vi "MainGui.vi"() -> ()   [LabVIEW 2016]
uses:
  MainGui.TestOptionsGui.ctl
  MainGui.TopBar.ctl
  tools/TouchPanel/TouchPanel.Keyboard.ctl
  tools/EventLog/EventLog.Gui.Sets.ctl
  tools/EventLog/EventLog.EventLevelOperatorGui.ctl
  MainGui.Action.ctl
  Sequence/Sequence.MainMode.ctl
  Station/Station.SwButtons.Fglb.Action.ctl
  Sequence/Sequence.UserAction.ctl
  MainGui.UserMsg.ctl
  tools/Translator/Translator.Message.ctl
  <vilib>/Utility/miscctls.llb/LVRowAndColumnTypeDef.ctl
  <vilib>/Utility/miscctls.llb/LVRowAndColumnUnsignedTypeDef.ctl
  tools/User/User.Level.ctl
  tools/CitTemplate/citTemplate.errData.ctl
  tools/EventLog/EventLog.EventSource.ctl
  Drivers/FestoCPX/FestoCPX.State.ctl
  Drivers/V7310/V7310.Data.Status.State.ctl
  Drivers/Keyence/Keyence.Data.Status.State.ctl
  tools/Translator/Translator.FormatMessage.vi
  tools/Config/Config.Global.vi
  Global/ApplicationGlobal.vi
  Station/Station.Global.vi
  tools/Translator/Translator.Global.vi
  Drivers/Keyence/LowLevel/Keyence.Global.vi
  Drivers/FestoCPX/FestoCPX.Global.vi
  Drivers/V7310/LowLevel/V7310.Global.vi
  <vilib>/Utility/inputDevices.llb/closeMouse.vi
  tools/User/User.Global.vi
  Database/Database.Global.vi
  MainGui.ButtonType.ctl
  <vilib>/Utility/miscctls.llb/LVRectTypeDef.ctl
panel:
  in  "Btn_ScannerGui":bool
  in  "Btn_Stats":bool
  in  "Btn_SelectPlate":bool
  in  "Btn_Scan":bool
  in  "Btn_DoorLock":bool
  in  "Btn_Reject":bool
  in  "Btn_Start":bool
  in  "Btn_ManualView":bool
  in  "Btn_Lock":bool
  in  "Btn_Pause":bool
  in  "Btn_Results":bool
  in  "Btn_Accept":bool
  in  "Btn_Next":bool
  in  "Btn_Exit":bool
  in  "Btn_Order":bool
  in  "Btn_Logs":bool
  in  "Btn_Base":bool
  in  "Btn_Manual":bool
  in  "Btn_Process":bool
  in  "Btn_Stop":bool
  in  "Btn_Mode":bool
  out "~ModeInUse":bool
  in  "EmptyButtons":bool[](array[boolean])
  out "Panel":refnum<vi>
  out "SelectModeTS":timestamp
  out "BlinkIndicator":bool
  out "RefNoTimer":timestamp
  out "Btns":refnum<vi>[](array[refnum])
  in  "TopBarTab":enum32{"Status", "Manual", "Logs", "Error"}(tab)=enum."Logs"
  out "StatusMsg":string
  in  "TestOptions":T1
  in  "EventModeOptions":T2={"IncludeBegin"=FALSE, "dtm_Begin"=timestamp(0 s since 1904-01-01), "IncludeEnd"=FALSE, "dtm_End"=timestamp(0 s since 1904-01-01), "Events Level Operator"=enum.">=", "Level"=1, "Source"=1, "SearchText"="", "Freeze"=FALSE} caption="Event.Sets" {"Source" items=["All", "Gui", "Ref", "File", "Arch", "Seq", "CPX", "DB", "Laser", "Scan.P", "Scan.O"]; "Level" items=["ALL", "Debug", "Info", "Warning", "Błąd"]; "dtm_End" format="%<%.1X\n%x>T"; "dtm_Begin" format="%<%.1X\n%x>T"}
  out "ErrMsg":i32(listbox)
  in  "Btn_ErrConfirm":bool
  in  "TopBar":T4={"~touchpanel"=FALSE, "_loop"=4, "_ver"="", "_flag"=bytes[0], "time"="", "Btn_ShowErr"=FALSE, "DB"=FALSE, "CPX"=FALSE, "LSR"=FALSE, "SCAN"=FALSE, "SCAN 2"=FALSE}
  in  "start here":bool
  out "MainPanelViRef":refnum<vi>
  out "DeviceID":refnum<k1> caption="device ID"
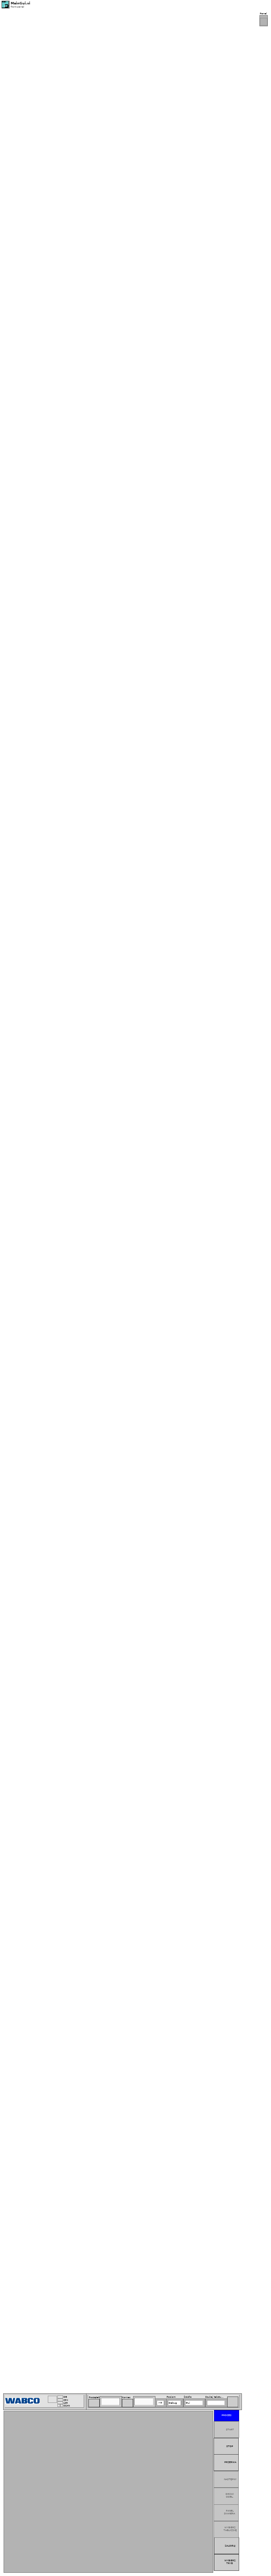
[diagram p1: front panel]
types:
  T1 = typedef "MainGui.TestOptionsGui.ctl" = cluster{"IgnoreResults":bool, "IgnoreImages":bool, "Service":bool}
  T2 = typedef "EventLog.Gui.Sets.ctl" = cluster{"IncludeBegin":bool, "dtm_Begin":timestamp, "IncludeEnd":bool, "dtm_End":timestamp, "Events Level Operator":T3, "Level":u16, "Source":u16, "SearchText":string, "Freeze":bool}
  T3 = typedef "EventLog.EventLevelOperatorGui.ctl" = enum16{">=", "=", "<="}
  T4 = typedef "MainGui.TopBar.ctl" = cluster{"~touchpanel":T5, "_loop":i32, "_ver":string, "_flag":picture, "time":string, "Btn_ShowErr":bool, "DB":bool, "CPX":bool, "LSR":bool, "SCAN":bool, "SCAN 2":bool}
  T5 = typedef "TouchPanel.Keyboard.ctl" = bool
  T6 = enum8{"Enabled", "Disabled", "Disabled and Grayed Out"}
  T7 = typedef "Translator.Message.ctl" = enum16{"-", "Event confirmed", "Log out", "Log in", "Shutdown", "Cancel", "Start", "Begin time", "End time", "Duration", "Service Mode", "Ignore Results", "Serial Format", "On", "Off", "OK", "NOK", "NOK %s", "Home", "Work", "Close", "Open", "In progress...", "Missing", "Empty", "Hardware failure", "Initial", "Default", "Total", "Out of range", "Free disk space is below 1GB - contact technician", "Error %d >> %s", "Error %d >> %s >> %s", "Msg %d >> %s", "Laser msg %d %s", "Laser cmd error %s %d", "Laser cmd failed %s", "Laser cmd warning %s", "Laser disconnected", "Laser status %s", "Laser already started", "Laser job unkonwn %s", "Laser job missing %s", "Laser job select failure %s", "Unable to start laser printing (%s)", "Unable to stop laser printing (%s)", "Laser marking aborted", "Laser marking timeout", "Unable to reset Laser Interlock (%s)", "Unable to trigger Laser. Laser not ready (%s)", "Laser job '%s' coordinates not configured", "Starting %s", "Quitting %s", "Configured", "Initializing", "Quitting", "Loading", "Loaded %d results", "Loaded %d events", "Running", "Stopped", "Summary", "Laser", "Do you want to continue?", "Do you want to delete the configuration?", "The configuration is being used by an order. Unable to delete!", "Press confirm button", "Station is not based. Do you want to exit?", "Station requires changeover. Do you want to run the test?", "Test options are not set as default. Do you want to continue?", "Formatting of WabcoNo is disabled. Do you want to continue?", "Product not detected. Do you want to continue?", "Product scan failed. Do you want to continue?", "Calibration", "Log out?", "System", "All", "IDLE", "Translating...%s", "Not found", "Alarm %s", "Run", "Skip", "Abort", "Repeat", "Please wait...", "Database disconnected", "Database disconnected - changeover disabled!", "Login to database successful", "Login to database failed: %d; %s", "Unable to check the product status of reference %d - database disconnected", "Unable to set the product status of reference %d - database disconnected", "Variant file backup %s", "Read variant (%s)", "Result", "Station armed!", "Station requires changeover!", "Select reference number...", "EMERGENCY BUTTON - press Control button", "EMERGENCY DOOR - press Control button", "Resetting Emergency...", "Unable to reset safety circuit - Emergency Button pressed", "Unable to reset safety circuit - Emergency Side Door open", "Station not based", "Station based", "Station not empty", "Station basing...", "No order", "Press Start to begin new order", "Scanning new order", "Order NOK. Correct or scan again", "Order OK. Press Accept", "Order ready", "Revolver incorrect", "Fork incorrect", "Revolver missing", "Revolver empty", "Container missing", "Offline results", "Offline statistics", "Updating statistics %.1f %%", "DMC Configurator", "Door open", "Close the front door", "Press start button", "Done. Open the front door", "Running...", "Running...%.1f %%", "Pause %s", "Pause %s. NOK container missing", "Pause %s. OK container missing", "Pause %s. Revolver empty", "Pause %s. Revolver missing", "Pause %s. Revolver incorrect", "Pause %s. Fork missing", "Pause %s. Fork incorrect", "Pause %s. Too many failures", "Pause %s. Unloading failure", "Pause %s. One slot is not working", "Pause %s. Part order is done. Empty OK container", "Pause %s. Unable to move product to slot", "Pause %s. Unable to move back product pusher", "Pause %s. Unable to lift product", "Pause %s. Unable to move back product lifter", "Pause %s. Unable to move product arm to Work", "Pause %s. Unable to move product arm to NOK", "Pause %s. Unable to move product arm to OK", "Pause %s. Unable to unsuck the NOK product", "Pause %s. Unable to drop the NOK product", "Pause %s. Product OK missing", "Pause %s. Unable to unsuck the OK product", "Pause %s. Unable to drop the OK product", "Stopping...", "File '%s' is missing", "File '%s' is broken", "File '%s' is running", "Log file started (%s)", "Log file ended (%s)", "Log file stopped (%s)", "Log file ignored (%s)", "Log file exported (%s)", "Log file export failed (%s)", "Wrong serial number in log file", "Wrong reference number in log file", "Test steps are missing", "%s = %.3f", "Process param '%s' not found in DB", "Process param '%s' wrong order", "Process param '%s' value %.3f out of limits (%.3f; %.3f)", "Step%d param '%s' not found in DB", "Step%d param '%s' wrong order", "Step%d param '%s' value %.3f out of limits (%.3f; %.3f)", "Step%d EV '%s' not found in DB", "Step%d EV '%s' wrong order", "\"%s\" not found in DB", "\"%s\" wrong order", "\"%s\" value %.3f out of limits (%.3f; %.3f)", "\"%s\" not found in software", "Process init (%s)", "Process started", "Process restarted", "Process run", "Process done", "Process done - remove OK container", "Process aborted", "Process aborted at work", "Process aborted at home", "Process error", "Process error at home", "Process error at work", "Process close", "Process pause", "Process continue", "Process door open", "Process door close", "Process pause at slot %s due to %s", "Select plate from the order to process", "Do you want to start the process?", "Do you want to continue the process?", "There is unfinished order. Do you want to put the new order?", "Product %s %d OK", "Product %s %d NOK", "Unable to unload the slot %s. Product missing in the slot", "Unable to unload the slot %s. Product already in the arm", "Unable to accept the product as OK. Product missing in slot %s", "Unable to accept the product as OK. Product could not drop into the container at slot %s", "Unable to accept the product as NOK. Product could not drop into the container at slot %s", "Scan failed. Error %s", "Scan failed. Scanner disconnected", "Scan failed. Wrong Wabco number %d, limit (%d,%d)", "Scan failed. Wrong serial number %d, limit (%d,%d)", "Scan failed. Wrong date %d, limit (%d,%d)", "Scan failed. Wrong product wabco number %d (expected %d)", "Scan failed. Wrong product serial number %d (expected > 0)", "Scan OK %s", "Scan failed. Unable to determine table position (%s)", "Scan failed. Timeout", "Tune failed. Scanner disconnected", "Tune failed. Timeout", "%s = %d", "%s = %d->%d", "Unable to set %s = %.2f - Air Pressure Inside off", "Unable to set digital output '%s' = %d", "Unable to activate air pressure inside - timeout", "Unable to activate air pressure inside - aborted", "Unable to switch on Air Main Valve - Air Pressure Inlet off", "Unable to switch on Air Main Valve - Door open", "Unable to switch off Air Main Valve - timeout", "Unable to switch off Air Main Valve - aborted", "Unable to rotate Table - timeout", "Unable to rotate Table - aborted", "Unable to rotate Table - Product Move not in Home position", "Unable to rotate Table - Air Pressure Inside off", "Unable to rotate Table - Product Lift A not in Home position", "Unable to rotate Table - Product Lift B not in Home position", "Unable to rotate Table - unlock before movement timeout", "Unable to rotate Table - lock after movement timeout", "Unable to move Table Lock to %s position - timeout", "Unable to move Table Lock to %s position - aborted", "Unable to move Table Lock to %s position - Air Pressure Inside off", "Unable to move Table Lock to %s position - Table not in position", "Unable to move Product Lift A to %s position - timeout", "Unable to move Product Lift B to %s position - timeout", "Unable to move Product Lift A to %s position - aborted", "Unable to move Product Lift B to %s position - aborted", "Unable to move Product Lift A to %s position - Air Pressure Inside off", "Unable to move Product Lift B to %s position - Air Pressure Inside off", "Unable to move Product Lift A to %s position - Table not locked", "Unable to move Product Lift B to %s position - Table not locked", "Unable to move Product Lift A to %s position - Product Arm not in Work position", "Unable to move Product Lift B to %s position - Product Arm not in Work position", "Unable to set Product Suction Gripper %s to %s - timeout", "Unable to set Product Suction Gripper %s to %s - aborted", "Unable to set Product Suction Gripper %s to %s - Air Pressure Inside off", "Unable to set Product Suction Gripper %s to %s - Table slot unkown", "Unable to move Product Arm to %s position - timeout", "Unable to move Product Arm to %s position - aborted", "Unable to move Product Arm to %s position - Air Pressure Inside off", "Unable to move Product Arm to %s position - Product Lift A not in Home position", "Unable to move Product Arm to %s position - Product Lift B not in Home position", "Unable to move Product to %s position - timeout", "Unable to move Product to %s position - aborted", "Unable to move Product to %s position - Air Pressure Inside off", "Unable to move Product to %s position - Table not in position"}
  T8 = typedef "Sequence.MainMode.ctl" = enum16{"Process", "Base", "Order", "Manual", "Logs", "Results", "Stats", "DMC Config"}
  T9 = typedef "Station.SwButtons.Fglb.Action.ctl" = enum16{"get", "start", "stop", "control"}
  T10 = typedef "Sequence.UserAction.ctl" = enum16{"-", "Stop", "Pause", "Continue", "Next"}
  T11 = typedef "LVRectTypeDef.ctl" = cluster{"Left":i16, "Top":i16, "Right":i16, "Bottom":i16}
  T12 = enum32{"Invalid", "Standard", "Closed", "Hidden", "Minimized", "Maximized"}
  T13 = typedef "MainGui.UserMsg.ctl" = cluster{"Msg":T7, "Arguments":variant[], "BgColor":u32, "TxtColor":u32, "Blink":bool}
  T14 = enum32{"invalid app kind", "Development System", "Run Time System", "Student Edition", "Embedded LabVIEW", "Evaluation", "Custom"}
  T15 = typedef "LVRowAndColumnUnsignedTypeDef.ctl" = cluster{"Row":u32, "Column":u32}
  T16 = typedef "LVRowAndColumnTypeDef.ctl" = cluster{"Row":i32, "Column":i32}
  T17 = typedef "User.Level.ctl" = enum16{"-", "Operator", "Technician", "Administrator"}
  T18 = typedef "citTemplate.errData.ctl" = cluster{"ts":timestamp, "src":T19, "instance":i32, "action":string, "error":errorcluster, "unconfirmed":bool}
  T19 = typedef "EventLog.EventSource.ctl" = enum16{"All", "Gui", "Ref", "File", "Arch", "Seq", "CPX", "DB", "Laser", "Scan.P", "Scan.O"}
  T20 = typedef "Keyence.Data.Status.State.ctl" = enum16{"First", "Init", "Reset", "Idle", "Scan", "Tune"}
  T21 = typedef "V7310.Data.Status.State.ctl" = enum16{"First", "Init", "Msg", "Error", "Abort", "Idle", "Run"}
  T22 = typedef "FestoCPX.State.ctl" = enum16{"First", "Error", "Init", "Run"}
  T23 = typedef "MainGui.Action.ctl" = enum32{"idle", "constructor", "destructor", "--- MainGui ---", "Error.Update", "Error.Confirm", "Buttons.Update", "Mode.Select", "Mode.Select.Seq", "Status.Update", "TopBar.Update"}
  T24 = typedef "Station.Data.ctl" = cluster{"State":T25, "Seq.State":T26, "Seq.BreakReason":T27, "Seq.BreakSource":T28, "Hw failure":bool, "Unconfirmed":bool, "Station empty":bool, "Home err":bool, "Order done":bool, "DUT present":T29, "EmgState":T30, "Sets":T31, "StatusBits":T33}
  T25 = typedef "Station.State.ctl" = enum16{"Idle", "Ready", "Run", "Stop", "Error", "Home", "Done", "Emg"}
  T26 = typedef "Sequence.State.ctl" = enum16{"Init", "Idle", "Home", "Work", "Run", "Pause"}
  T27 = typedef "Sequence.Test.BreakReason.ctl" = enum16{"-", "NOK container", "OK container", "Rev empty", "Rev missing", "Rev wrong", "Fork missing", "Fork wrong", "NOK limit", "Unload failure", "Single slot", "Part done", "Err: Prod move work", "Err: Prod move home", "Err: Prod lift work", "Err: Prod lift home", "Err: Prod Arm Work", "Err: Prod Arm NOK", "Err: Prod Arm OK", "Err: Prod NOK suck", "Err: Prod NOK drop", "Err: Prod OK missing", "Err: Prod OK suck", "Err: Prod OK drop"}
  T28 = typedef "Sequence.Test.BreakSource.ctl" = enum16{"-", "A", "B", "A/B"}
  T29 = typedef "FestoCPX.Station.ProdPresent.ctl" = cluster{"Slot1":cluster{"A":bool, "B":bool}, "Slot2":cluster{"A":bool, "B":bool}, "Slot3":cluster{"A":bool, "B":bool}, "Slot4":cluster{"A":bool, "B":bool}, "Final":cluster{"A":bool, "B":bool}, "OK":cluster{"A":bool, "B":bool}, "Container":cluster{"OK":bool, "NOK":bool}}
  T30 = typedef "FestoCPX.Station.EmgState.ctl" = cluster{"Button":bool, "SideDoor":bool, "FrontDoor":bool, "DoorSecured":bool}
  T31 = typedef "Sequence.UserData.ctl" = cluster{"GuiMode":T8, "Test":T32, "ContinueOrder":bool}
  T32 = typedef "MainGui.TestOptions.ctl" = cluster{"IgnoreResults":bool, "IgnoreImages":bool, "ServiceMode":bool}
  T33 = typedef "Station.Home.Status.Bits.ctl" = cluster{"Door Close":bool, "Rev OK":bool, "Fork OK":bool, "Container OK":bool, "Station empty":bool}
  T34 = typedef "Sequence.PlateType.ctl" = enum16{"Wabco", "Client"}
  T35 = typedef "LVPositionTypeDef.ctl" = cluster{"Left":i32, "Top":i32}
  T36 = typedef "Keyence.Data.Status.ctl" = cluster{"State":T20, "Ref":refnum<k5>, "Bank":u8, "Version":string, "Model":string, "EndTS":timestamp, "ImgPath":path, "Tuned":bool}
  T37 = typedef "FestoCPX.Data.Status.ctl" = cluster{"State":T22, "Conn":refnum<k5>, "TS":timestamp}
  T38 = typedef "V7310.Data.Status.ctl" = cluster{"State":T21, "LaserStatus":T39, "LaserStatusRaw":string, "Ref":refnum<k5>, "RTC TS":timestamp, "Conn TS":timestamp, "Msg":T40[], "JobInUse":string, "Jobs":string[], "Vars":T41[]}
  T39 = typedef "V7310.LaserStatus.ctl" = enum16{"-", "FatalError", "Initialize", "KeySwitchOpen", "TimeoutInterlock", "InterlockOpen", "StartUp", "ShutterlockOpen", "Standby", "Ready", "PrepareForMarking", "WaitForTrigger", "Marking"}
  T40 = typedef "V7310.Message.Data.ctl" = cluster{"ID":i32, "Msg":string}
  T41 = typedef "V7310.Job.Variable.ctl" = cluster{"Name":string, "Value":string}
  T42 = typedef "Database.Main.Data.Status.ctl" = cluster{"Run":bool, "Handle":i32, "ConnTS":timestamp, "DbTime":timestamp, "DbTimeCode":dbl, "DbTimeOffset":dbl}
  T43 = typedef "MainGui.ButtonType.ctl" = enum32{"Exit", "Mode", "Process", "Base", "Order", "Manual", "Logs", "Results", "Accept", "Reject", "Start", "Stop", "Next", "Pause", "Lock", "ManualView", "DoorLock", "Scan", "Select", "ScannerGui", "Stats"}
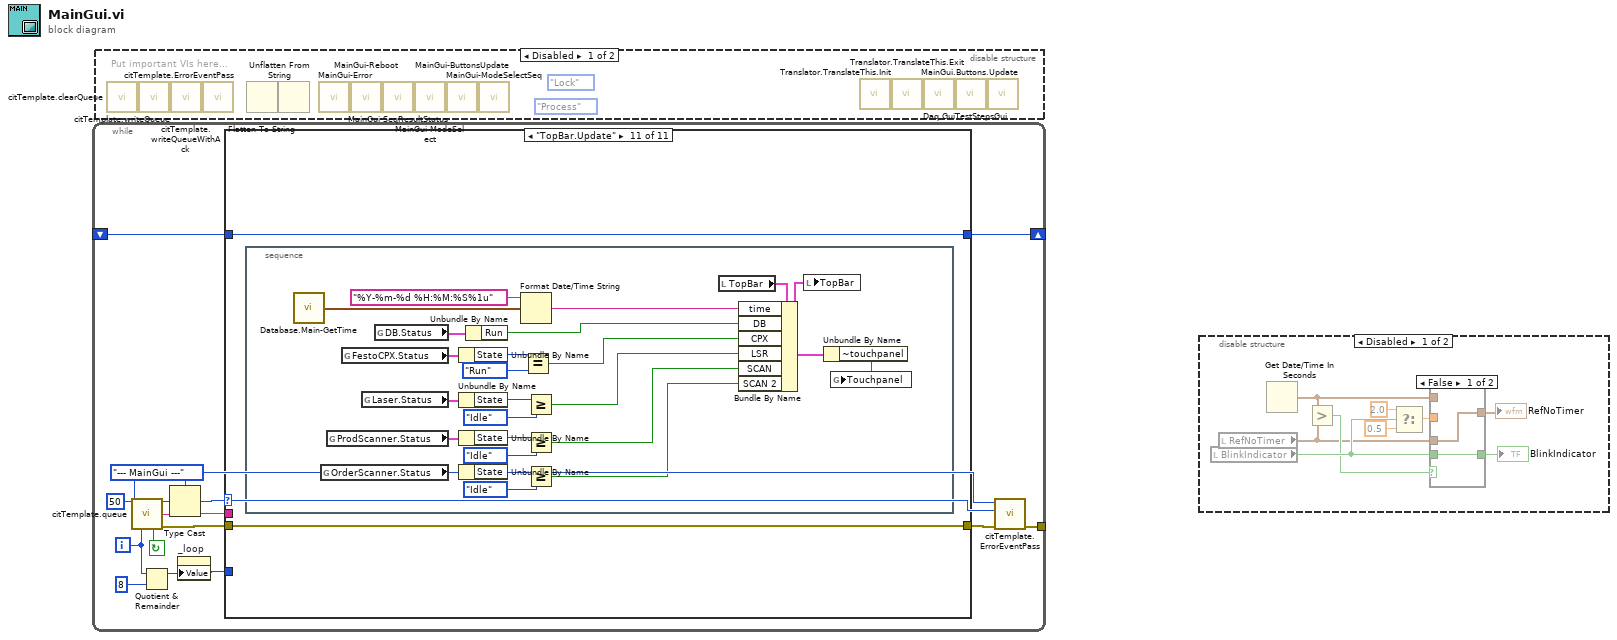
[diagram p0: block diagram]
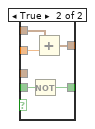
[diagram p2: hidden frame]
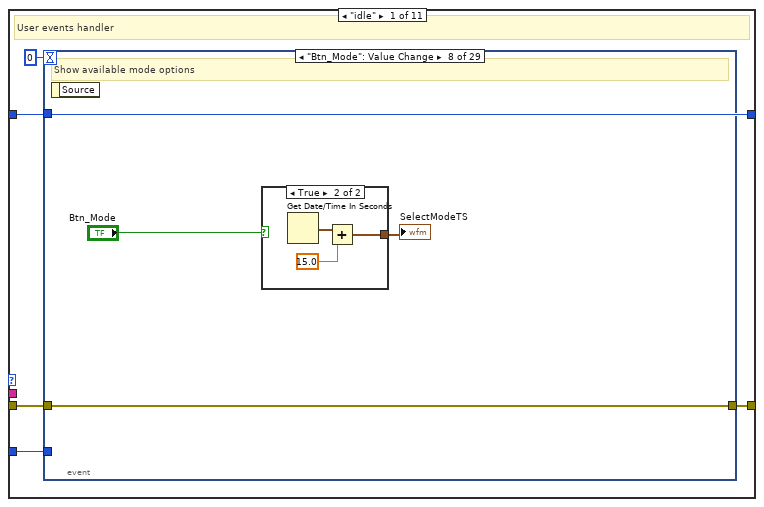
[diagram p5: hidden frame]
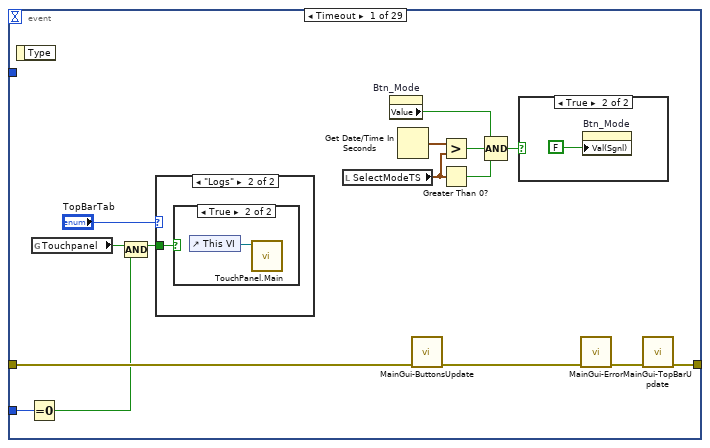
[diagram p6: hidden frame]
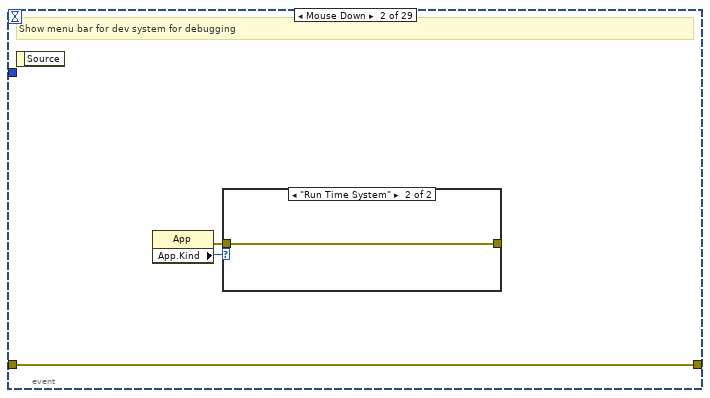
[diagram p10: hidden frame]
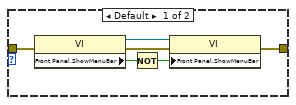
[diagram p11: hidden frame]
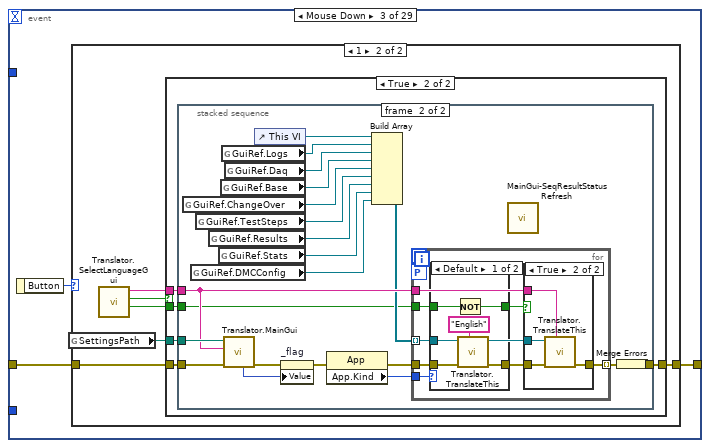
[diagram p12: hidden frame]
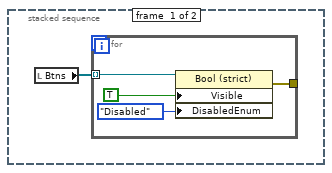
[diagram p15: hidden frame]
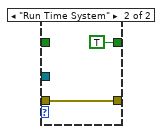
[diagram p17: hidden frame]
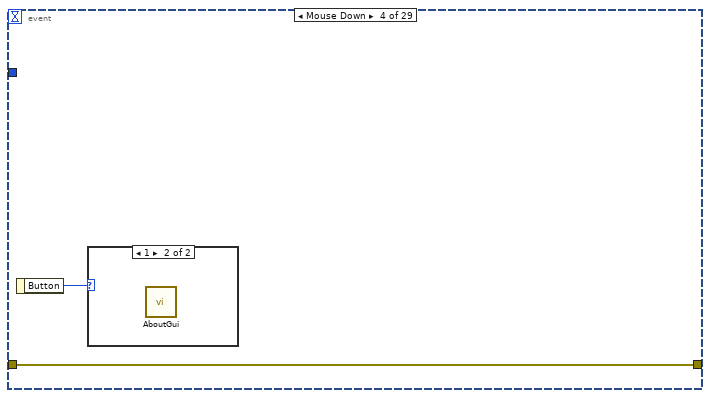
[diagram p18: hidden frame]
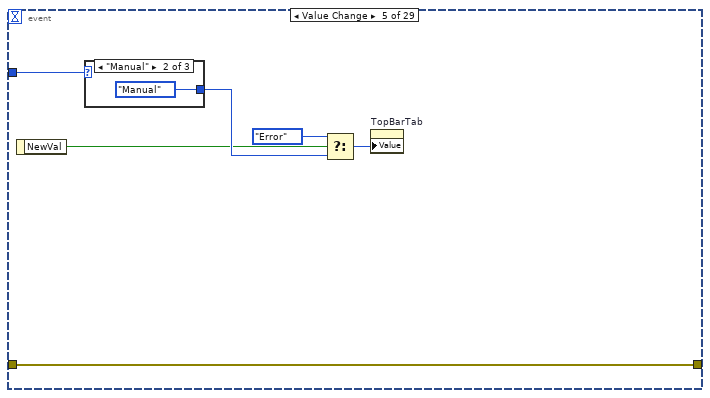
[diagram p20: hidden frame]
diagram:
  n1 = while {
    tunnel: [w7] -> _
    shift-right: [w2] -> _
    shift-left: _ -> [w4]
    i -> [w8]
    stop <- w11 continue-if-true
    w10 = MainGui.Action."--- MainGui ---" ("Action")
    n2 = call "citTemplate.queue.vi"("ms timeout (250 ms)"=50, "event enum"=w10, "iteration (-1)"=w8) -> ("event out"=w14:u32, "(flatten) data out"=w13:string, "continue"=w11:bool, "error out"=w12:errorcluster)  [unwired: 2 in, 7 out]
    n3 = Quotient & Remainder(x=w8, y=8) -> (x-y*floor(x/y)=w1:i32)  [unwired: 1 out]
    n4 = Type Cast(type=w10, x=w14) -> (*(type *) &x=w6:T23)
    n5 = property on="_loop" class="Ring (strict)"("Value"=w1) -> ()  [unwired: 2 in, 2 out]
    n6 = case shown="\"TopBar.Update\"" w6 {
      selector: w6 -> [_ _ _ w381 _ _ _ _ _ _ _]
      tunnel: w13 -> [_ _ _ w382 _ _ _ w444 _ w537 _]
      tunnel: w12 -> [w19 w247 w336 w384 w396 w426 w434 w445 w515 w538 w547]
      tunnel: w4 -> [w16 _ w334 w380 w393 w427 w437 w439 w516 w539 w548]
      tunnel: [w16 w246 w334 w380 w393 w427 w437 w440 w516 w539 w548] -> w2
      tunnel: [w18 w245 w335 w373 w397 w425 w432 w441 w510 w535 w547] -> w3
      tunnel: w1 -> [w15 _ _ _ _ _ _ _ _ _ _]
      frame "idle" {
        # "User events handler"
        n7 = event shown="[7] \"Btn_Mode\": Value Change" {
          selector: _ -> [_ _ _ _ _ _ _ _ _ _ _ _ _ _ _ _ _ _ _ _ _ _ _ _ _ _ _ _ _]
          dyn-events: _ -> [_ _ _ _ _ _ _ _ _ _ _ _ _ _ _ _ _ _ _ _ _ _ _ _ _ _ _ _ _]
          timeout: 0 -> [_ _ _ _ _ _ _ _ _ _ _ _ _ _ _ _ _ _ _ _ _ _ _ _ _ _ _ _ _]
          tunnel: w19 -> [w34 w40 w49 w112 w115 w124 w126 w146 w152 w155 w158 w161 w164 w167 w169 w173 w188 w196 w198 w201 w207 w209 w213 w214 w220 w237 w240 w242 w244]
          tunnel: [w33 w40 w48 w112 w115 w124 w125 w146 w151 w154 w156 w160 w163 w166 w168 w172 w186 w196 w197 w201 w206 w208 w212 w214 w220 w237 w239 w241 w244] -> w18
          tunnel: w16 -> [_ _ _ _ w118 _ _ _ _ _ _ _ _ _ _ w171 w187 _ _ _ _ _ _ _ w218 _ _ _ _]
          tunnel: w15 -> [w23 _ _ _ _ _ _ _ _ _ _ _ _ _ _ _ _ _ _ _ _ _ _ _ _ _ _ _ _]
          event Timeout {
            n8 = event-data() -> ()  [unwired: 1 in, 1 out]
            n9 = Equal To 0?(x=w23) -> (x = 0?=w21:bool)
            n10 = global read "Config.Global.vi" "Touchpanel"() -> (w32:bool)
            n11 = Compound Arithmetic op=AND(w32, w21) -> (w22:bool)
            n12 = case shown="\"Logs\"" "TopBarTab" {
              tunnel: w22 -> [_ w35]
              frame Default {
              }
              frame "Logs" {
                n13 = case shown="True" w35 {
                  frame False {
                  }
                  frame True {
                    n14 = control-ref of="This VI"() -> (w36:refnum<vi>)
                    n15 = call "TouchPanel.Main.vi"("VI ref"=w36) -> ()  [unwired: 8 in, 3 out]
                  }
                }
              }
            }
            n16 = local read "SelectModeTS"() -> (w25:timestamp)
            n17 = property on="Btn_Mode" class="Bool (strict)"() -> ("Value"=w28:bool)  [unwired: 2 in, 2 out]
            n18 = Get Date/Time In Seconds() -> (seconds since 1Jan1904=w24:timestamp)
            n19 = call "MainGui-ButtonsUpdate.vi"("error in (no error)"=w34) -> ("error out"=w30:errorcluster)  [unwired: 10 in]
            n20 = Greater?(x=w24, y=w25) -> (0:w26:bool)
            n21 = Greater Than 0?(x=w25) -> (x > 0?=w27:bool)
            n22 = Compound Arithmetic op=AND(w28, w26, w27) -> (w29:bool)
            n23 = case shown="True" w29 {
              frame False {
              }
              frame True {
                n24 = property on="Btn_Mode" class="Bool (strict)"("Val(Sgnl)"=FALSE ("Value (Signaling)")) -> ()  [unwired: 2 in, 2 out]
              }
            }
            n25 = call "MainGui-Error.vi"("error in (no error)"=w30) -> ("error out"=w31:errorcluster)  [unwired: 10 in]
            n26 = call "MainGui-TopBarUpdate.vi"("error in (no error)"=w31) -> ("error out"=w33:errorcluster)  [unwired: 10 in]
          }
          event Mouse Down {
            # "Show menu bar for dev system for debugging"
            n27 = event-data() -> ()  [unwired: 1 in, 1 out]
            n28 = property class="App"() -> (error out=w38:errorcluster, "App.Kind"=w39:T14)  [unwired: 2 in, 1 out]
            n29 = case shown="\"Run Time System\"" w39 {
              tunnel: w38 -> [w42 w47]
              tunnel: [w41 w47] -> _
              frame Default {
                n30 = property class="VI"(error in=w42) -> (reference out=w46:refnum<vi>, error out=w45:errorcluster, "Front Panel.ShowMenuBar"=w44:bool)  [unwired: 1 in]
                n31 = Not(x=w44) -> (.not. x?=w43:bool)
                n32 = property class="VI"(reference=w46, error in=w45, "Front Panel.ShowMenuBar"=w43) -> (error out=w41:errorcluster)  [unwired: 1 out]
              }
              frame "Run Time System" {
              }
            }
          }
          event Mouse Down {
            n33 = event-data() -> ("Button"=w50:u16)  [unwired: 1 in]
            n34 = case shown="1" w50 {
              tunnel: w49 -> [w51 w55]
              tunnel: [w51 w54] -> w48
              frame Default {
              }
              frame 1 {
                n35 = global read "ApplicationGlobal.vi" "SettingsPath"() -> (w52:path)
                n36 = call "Translator.SelectLanguageGui.vi"() -> ("english"=w56:bool, "changed"=w57:bool, "Language"=w53:string)  [unwired: 9 in]
                n37 = case shown="True" w57 {
                  tunnel: w56 -> [_ w60]
                  tunnel: w55 -> [w58 w63]
                  tunnel: [w58 w59] -> w54
                  tunnel: w53 -> [_ w61]
                  tunnel: w52 -> [_ w62]
                  frame False {
                  }
                  frame True {
                    n38 = stacked-sequence {
                      tunnel: w63 -> [_ w89]
                      tunnel: w62 -> [_ w88]
                      tunnel: w61 -> [_ w87]
                      tunnel: w60 -> [_ w77]
                      tunnel: [_ w76] -> w59
                      frame #0 {
                        n39 = local read "Btns"() -> (w64:refnum<vi>[])
                        n40 = for {
                          tunnel: w64 -> [w68] mode=indexing
                          tunnel: [w65] -> _
                          n41 = property class="Bool (strict)"(reference=w68, "Visible"=TRUE, "DisabledEnum"=T6."Disabled" ("Disabled")) -> (error out=w65:errorcluster)  [unwired: 1 in, 1 out]
                        }
                      }
                      frame #1 {
                        n42 = global read "ApplicationGlobal.vi" "GuiRef.ChangeOver"() -> (w79:refnum<vi>)
                        n43 = global read "ApplicationGlobal.vi" "GuiRef.DMCConfig"() -> (w69:refnum<vi>)
                        n44 = global read "ApplicationGlobal.vi" "GuiRef.TestSteps"() -> (w80:refnum<vi>)
                        n45 = global read "ApplicationGlobal.vi" "GuiRef.Results"() -> (w72:refnum<vi>)
                        n46 = global read "ApplicationGlobal.vi" "GuiRef.Stats"() -> (w70:refnum<vi>)
                        n47 = global read "ApplicationGlobal.vi" "GuiRef.Base"() -> (w81:refnum<vi>)
                        n48 = global read "ApplicationGlobal.vi" "GuiRef.Logs"() -> (w71:refnum<vi>)
                        n49 = call "Translator.MainGui.vi"("~error in"=w89, "~Language in use"=w87, "~Translation folder"=w88) -> ("~error out"=w75:errorcluster, "~flag small"=w73:picture)  [unwired: 5 in, 2 out]
                        n50 = global read "ApplicationGlobal.vi" "GuiRef.Daq"() -> (w82:refnum<vi>)
                        n51 = control-ref of="This VI"() -> (w83:refnum<vi>)
                        n52 = property on="_flag" class="Pict"(error in=w75, "Value"=w73) -> (error out=w74:errorcluster)  [unwired: 1 in, 1 out]
                        n53 = property class="App"(error in=w74) -> (error out=w84:errorcluster, "App.Kind"=w85:T14)  [unwired: 1 in, 1 out]
                        n54 = Build Array(w83, w71, w82, w81, w79, w80, w72, w70, w69) -> (w78:refnum<vi>[])
                        n55 = for {
                          tunnel: w87 -> [w97]
                          tunnel: w85 -> [w94]
                          workers-P: _ -> [_]
                          tunnel: w78 -> [w92] mode=indexing
                          tunnel: w77 -> [w91]
                          tunnel: w84 -> [w93]
                          tunnel: [w95] -> w86 mode=indexing
                          n56 = case shown="Default" w94 {
                            tunnel: [w107 w110] -> w96
                            tunnel: w93 -> [w106 w110]
                            tunnel: w92 -> [w105 _]
                            tunnel: w91 -> [w104 _]
                            tunnel: [w103 TRUE ("english")] -> w90
                            frame Default {
                              n57 = Not(x=w104) -> (.not. x?=w103:bool)
                              n58 = call "Translator.TranslateThis.vi"("Language (English)"="English" ("Language"), "error in"=w106, "vi reference"=w105) -> ("error out"=w107:errorcluster)  [unwired: 8 in]
                            }
                            frame "Run Time System" {
                            }
                          }
                          n59 = case shown="True" w90 {
                            tunnel: w97 -> [_ w102]
                            tunnel: w96 -> [w98 w101]
                            tunnel: [w98 w100] -> w95
                            tunnel: w92 -> [_ w99]
                            frame False {
                            }
                            frame True {
                              n60 = call "Translator.TranslateThis.vi"("Language (English)"=w102, "error in"=w101, "vi reference"=w99) -> ("error out"=w100:errorcluster)  [unwired: 8 in]
                            }
                          }
                        }
                        n61 = call "MainGui-SeqResultStatusRefresh.vi"() -> ()  [unwired: 11 in, 1 out]
                        n62 = Merge Errors(w86) -> (w76:errorcluster)
                      }
                    }
                  }
                }
              }
            }
          }
          event Mouse Down {
            n63 = event-data() -> ("Button"=w111:u16)  [unwired: 1 in]
            n64 = case shown="1" w111 {
              frame Default {
              }
              frame 1 {
                n65 = call "AboutGui.vi"() -> ()  [unwired: 12 in]
              }
            }
          }
          event Value Change {
            n66 = event-data() -> ("NewVal"=w116:bool)  [unwired: 1 in]
            n67 = case shown="\"Manual\"" w118 {
              tunnel: [enum32{"Status", "Manual", "Logs", "Error"}."Status" ("TopBarTab") enum32{"Status", "Manual", "Logs", "Error"}."Manual" ("TopBarTab") enum32{"Status", "Manual", "Logs", "Error"}."Logs" ("TopBarTab")] -> w117
              frame Default {
              }
              frame "Manual" {
              }
              frame "Logs" {
              }
            }
            n68 = Select(t=enum32{"Status", "Manual", "Logs", "Error"}."Error" ("TopBarTab"), s=w116, f=w117) -> (s? t:f=w113:enum32{"Status", "Manual", "Logs", "Error"})
            n69 = property on="TopBarTab" class="TabCtl (strict)"("Value"=w113) -> ()  [unwired: 2 in, 2 out]
          }
          event "Btn_ErrConfirm": Value Change {
            # "Confirm error"
            n70 = event-data() -> ()  [unwired: 1 in, 1 out]
            n71 = global read "Station.Global.vi" "Station"() -> (w123:T24)
            n72 = Unbundle By Name(w123) -> ("State"=w122:T25)
            n73 = case shown="Default" w122 {
              frame Default {
                n74 = call "ErrorHandling.Fglb.Confirm.vi"() -> ()  [unwired: 11 in, 1 out]
              }
              frame "Error" {
                n75 = call "Station-StatusClear.vi"() -> ()  [unwired: 11 in, 1 out]
              }
            }
          }
          event "Btn_Exit": Value Change {
            # "Exit application"
            n76 = event-data() -> ()  [unwired: 1 in, 1 out]
            n77 = disable-structure shown="Enabled" {
              disable-tunnel: [w132 TRUE ("ok")] -> w127
              frame Disabled {
                n78 = global read "Station.Global.vi" "Station"() -> (w131:T24)
                n79 = Unbundle By Name(w131) -> ("State"=w130:T25)
                n80 = call "Translator.Translate.Status (NoError).vi"("msg"=Translator.Message."Station is not based. Do you want to exit?") -> ("Translated Msg"=w128:string)  [unwired: 10 in]
                n81 = case shown="Default" w130 {
                  tunnel: [TRUE ("ok") w135] -> w132
                  tunnel: w128 -> [_ w134]
                  frame "Ready" {
                  }
                  frame Default {
                    n82 = call "ExitGui.vi"("Message"=w134) -> ("ok"=w135:bool)  [unwired: 9 in, 1 out]
                  }
                }
              }
              frame Enabled {
              }
            }
            n83 = stacked-sequence {
              tunnel: [w140] -> w125
              tunnel: w126 -> [w138]
              tunnel: w127 -> [w137]
              frame #0 {
                n84 = case shown="True" w137 {
                  tunnel: w138 -> [w141 w142]
                  tunnel: [w141 w143] -> w140
                  frame False {
                  }
                  frame True {
                    n85 = call "MainGui-Reboot.vi"("error in (no error)"=w142) -> ("error out"=w143:errorcluster)  [unwired: 10 in]
                  }
                }
                n86 = local write "Btn_Mode"(FALSE ("Btn_SelMode")) -> ()
              }
            }
          }
          event "Btn_Mode": Value Change {
            # "Show available mode options"
            n87 = event-data() -> ()  [unwired: 1 in, 1 out]
            n88 = case shown="True" "Btn_Mode" {
              tunnel: [_ w147] -> w145
              frame False {
              }
              frame True {
                n89 = Get Date/Time In Seconds() -> (seconds since 1Jan1904=w149:timestamp)
                n90 = Add(x=w149, y=15.0) -> (x+y=w147:timestamp)
              }
            }
            "SelectModeTS" <- w145
          }
          event "Btn_Process": Value Change {
            # "Enter mode: Auto"
            n91 = event-data() -> ()  [unwired: 1 in, 1 out]
            n92 = call "MainGui-ModeSelect.vi"("error in (no error)"=w152, "Mode"=Sequence.MainMode."Process") -> ("error out"=w151:errorcluster)  [unwired: 9 in]
          }
          event "Btn_Manual": Value Change {
            # "Enter mode: Manual"
            n93 = event-data() -> ()  [unwired: 1 in, 1 out]
            n94 = call "MainGui-ModeSelect.vi"("error in (no error)"=w155, "Mode"=Sequence.MainMode."Manual") -> ("error out"=w154:errorcluster)  [unwired: 9 in]
          }
          event "Btn_Base": Value Change {
            # "Enter mode: Base"
            n95 = event-data() -> ()  [unwired: 1 in, 1 out]
            n96 = call "MainGui-ModeSelect.vi"("error in (no error)"=w158, "Mode"=Sequence.MainMode."Base") -> ("error out"=w156:errorcluster)  [unwired: 9 in]
          }
          event "Btn_Order": Value Change {
            # "Enter mode: Rearming"
            n97 = event-data() -> ()  [unwired: 1 in, 1 out]
            n98 = call "MainGui-ModeSelect.vi"("error in (no error)"=w161, "Mode"=Sequence.MainMode."Order") -> ("error out"=w160:errorcluster)  [unwired: 9 in]
          }
          event "Btn_Logs": Value Change {
            # "Enter mode: Events"
            n99 = event-data() -> ()  [unwired: 1 in, 1 out]
            n100 = call "MainGui-ModeSelect.vi"("error in (no error)"=w164, "Mode"=Sequence.MainMode."Logs") -> ("error out"=w163:errorcluster)  [unwired: 9 in]
          }
          event "Btn_Results": Value Change {
            # "Enter mode: Events"
            n101 = event-data() -> ()  [unwired: 1 in, 1 out]
            n102 = call "MainGui-ModeSelect.vi"("error in (no error)"=w167, "Mode"=Sequence.MainMode."Results") -> ("error out"=w166:errorcluster)  [unwired: 9 in]
          }
          event "Btn_Stats": Value Change {
            n103 = event-data() -> ()  [unwired: 1 in, 1 out]
            n104 = call "MainGui-ModeSelect.vi"("error in (no error)"=w169, "Mode"=Sequence.MainMode."Stats") -> ("error out"=w168:errorcluster)  [unwired: 9 in]
          }
          event "Btn_Accept": Value Change {
            n105 = event-data() -> ()  [unwired: 1 in, 1 out]
            n106 = case shown="\"DMC Config\"" w171 {
              tunnel: w173 -> [w174 w176 w179]
              tunnel: [w174 w175 w180] -> w172
              frame Default {
              }
              frame "Order" {
                n107 = call "ChangeOverGui-RefAccept.vi"("error in"=w176) -> ("error out"=w175:errorcluster)  [unwired: 10 in]
              }
              frame "DMC Config" {
                n108 = global read "Config.Global.vi" "Password.DMCConfig"() -> (w178:string)
                n109 = call "LoginGui.vi"("Password"=w178) -> ("ok?"=w177:bool)  [unwired: 10 in]
                n110 = case shown="True" w177 {
                  tunnel: [w181 w185] -> w180
                  tunnel: w179 -> [w181 w183]
                  frame False {
                  }
                  frame True {
                    n111 = call "DMCConfiguratorGui-Accept.vi"("error in"=w183) -> ("error out"=w182:errorcluster)  [unwired: 10 in]
                    n112 = call "MainGui-ModeSelect.vi"("error in (no error)"=w182, "Mode"=Sequence.MainMode."Order") -> ("error out"=w185:errorcluster)  [unwired: 9 in]
                  }
                }
              }
            }
          }
          event "Btn_Reject": Value Change {
            n113 = event-data() -> ()  [unwired: 1 in, 1 out]
            n114 = case shown="\"DMC Config\"" w187 {
              tunnel: w188 -> [w189 w191 w194]
              tunnel: [w189 w190 w193] -> w186
              frame Default {
              }
              frame "Order" {
                n115 = call "ChangeOverGui-RefReject.vi"("error in"=w191) -> ("error out"=w190:errorcluster)  [unwired: 10 in]
              }
              frame "DMC Config" {
                n116 = call "MainGui-ModeSelect.vi"("error in (no error)"=w194, "Mode"=Sequence.MainMode."Order") -> ("error out"=w193:errorcluster)  [unwired: 9 in]
              }
            }
          }
          event "Btn_Start": Value Change {
            # "Start test sequence"
            n117 = event-data() -> ()  [unwired: 1 in, 1 out]
            n118 = call "Station.SwButtons.Fglb.vi"("action (get)"=Station.SwButtons.Fglb.Action."start") -> ()  [unwired: 1 in, 1 out]
          }
          event "Btn_Scan": Value Change {
            n119 = event-data() -> ()  [unwired: 1 in, 1 out]
            n120 = call "ChangeOverGui-Scan.vi"("error in"=w198) -> ("error out"=w197:errorcluster)  [unwired: 10 in]
          }
          event "Btn_Stop": Value Change {
            # "Stop test sequence"
            n121 = event-data() -> ()  [unwired: 1 in, 1 out]
            n122 = global write "Station.Global.vi" "ProcStop"(TRUE ("ProcStop")) -> ()
            n123 = call "Station.SwButtons.Fglb.vi"("action (get)"=Station.SwButtons.Fglb.Action."stop") -> ()  [unwired: 1 in, 1 out]
          }
          event "Btn_Pause": Value Change {
            n124 = event-data() -> ("NewVal"=w205:bool)  [unwired: 1 in]
            n125 = Select(t=Sequence.UserAction."Pause" ("UserAction"), s=w205, f=Sequence.UserAction."Continue" ("UserAction")) -> (s? t:f=w202:T10)
            n126 = call "Sequence-UserAction.vi"("error in (no error)"=w207, "UserAction"=w202) -> ("error out"=w206:errorcluster)  [unwired: 9 in]
          }
          event "Btn_Next": Value Change {
            # "Step mode: Run the next step"
            n127 = event-data() -> ()  [unwired: 1 in, 1 out]
            n128 = call "Sequence-UserAction.vi"("error in (no error)"=w209, "UserAction"=Sequence.UserAction."Next") -> ("error out"=w208:errorcluster)  [unwired: 9 in]
          }
          event "Btn_DoorLock": Value Change {
            # "Step mode: Run the next step"
            n129 = event-data() -> ()  [unwired: 1 in, 1 out]
            n130 = call "Sequence-DoorLock.vi"("error in (no error)"=w213, "Door Lock State"="Btn_DoorLock") -> ("error out"=w212:errorcluster)  [unwired: 9 in]
          }
          event "Btn_SelectPlate": Value Change {
            n131 = event-data() -> ()  [unwired: 1 in, 1 out]
            n132 = call "ProcessInfoGui.vi"() -> ("cancel"=w216:bool, "PlateType"=w215:T34)  [unwired: 10 in]
            n133 = case shown="False" w216 {
              tunnel: w215 -> [w217 _]
              frame False {
                n134 = call "Sequence-SelectPlate.vi"("PlateType"=w217) -> ()  [unwired: 10 in, 1 out]
              }
              frame True {
              }
            }
          }
          event "Btn_Lock": Value Change {
            n135 = event-data() -> ()  [unwired: 1 in, 1 out]
            n136 = case shown="\"DMC Config\"" w218 {
              tunnel: "Btn_Lock" -> [w223 w233]
              frame "DMC Config" {
                n137 = global read "Config.Global.vi" "Password.DMCConfig"() -> (w222:string)
                n138 = case shown="True" w223 {
                  tunnel: [_ w225] -> w221
                  tunnel: w222 -> [_ w224]
                  frame False {
                  }
                  frame True {
                    n139 = call "LoginGui.vi"("Password"=w224) -> ("ok?"=w225:bool)  [unwired: 10 in]
                  }
                }
                n140 = global write "ApplicationGlobal.vi" "DMCConfig.Unlock"(w221) -> ()
              }
              frame Default {
                n141 = global read "Config.Global.vi" "Password"() -> (w226:string)
                n142 = case shown="True" w233 {
                  tunnel: [_ w235] -> w232
                  tunnel: w226 -> [_ w234]
                  frame False {
                  }
                  frame True {
                    n143 = call "LoginGui.vi"("Password"=w234) -> ("ok?"=w235:bool)  [unwired: 10 in]
                  }
                }
                n144 = global write "ApplicationGlobal.vi" "Unlock"(w232) -> ()
                n145 = Select(t=T6."Enabled" ("Disabled"), s=w232, f=T6."Disabled and Grayed Out" ("Disabled")) -> (s? t:f=w227:T6)
                n146 = property on="IgnoreResults" class="Bool (strict)"("DisabledEnum"=w227) -> (error out=w229:errorcluster)  [unwired: 2 in, 1 out]
                n147 = property on="IgnoreImages" class="Bool (strict)"(error in=w229, "DisabledEnum"=w227) -> (error out=w228:errorcluster)  [unwired: 1 in, 1 out]
                n148 = property on="Service" class="Bool (strict)"(error in=w228, "DisabledEnum"=w227) -> ()  [unwired: 1 in, 2 out]
              }
            }
          }
          event "Btn_ManualView": Value Change {
            n149 = event-data() -> ()  [unwired: 1 in, 1 out]
            n150 = global write "ApplicationGlobal.vi" "ManualView"("Btn_ManualView") -> ()
          }
          event "Btn_ScannerGui": Value Change {
            n151 = event-data() -> ()  [unwired: 1 in, 1 out]
            n152 = call "Keyence.Gui.vi"("error in"=w240, "Idx"=0) -> ("error out"=w239:errorcluster)  [unwired: 9 in]
          }
          event Value Change {
            n153 = event-data() -> ()  [unwired: 1 in, 1 out]
            n154 = call "MainGui-ModeSelectSeq.vi"("error in (no error)"=w242) -> ("error out"=w241:errorcluster)  [unwired: 10 in]
          }
          event Value Change {
            n155 = event-data() -> ()  [unwired: 1 in, 1 out]
            n156 = global write "Config.Global.vi" "LogsOptions"("EventModeOptions") -> ()
          }
        }
      }
      frame "constructor" {
        # "Application initialization actions"
        n157 = stacked-sequence {
          tunnel: w247 -> [_ _ _ _ _ _ w329 _]
          tunnel: [_ _ _ _ _ _ Sequence.MainMode."Process" ("f") _] -> w246
          tunnel: [_ _ _ _ _ _ w324 _] -> w245
          frame #0 {
            # "Init FP"
            n158 = property on="start here" class="Bool (strict)"() -> (error out=w255:errorcluster, "Position"=w254:T35)  [unwired: 2 in, 1 out]
            n159 = property on="Pane" class="Pane"(error in=w255, "Origin"=w254, "PaneColor"=u32 16777226) -> (error out=w253:errorcluster)  [unwired: 1 in, 1 out]
            n160 = disable-structure shown="Enabled" {
              disable-tunnel: w253 -> [w259 w263]
              disable-tunnel: [w257 w261] -> w249
              frame Disabled {
                n161 = property class="VI"(error in=w259, "FP.State"=T12."Standard" ("Front Panel Window:State"), "Front Panel.ShowMenuBar"=FALSE ("Front Panel Window:Show Menu Bar"), "Front Panel.PanelBounds"=T11 {"Left"=0, "Top"=0, "Right"=1024, "Bottom"=768} ("Front Panel Window:Panel Bounds")) -> ("Panel"=w257:refnum<vi>)  [unwired: 1 in, 2 out]
              }
              frame Enabled {
                n162 = property class="VI"(error in=w263, "FP.State"=T12."Standard" ("Front Panel Window:State"), "Front Panel.ShowMenuBar"=FALSE ("Front Panel Window:Show Menu Bar")) -> ("Panel"=w261:refnum<vi>)  [unwired: 1 in, 2 out]
              }
            }
            "Panel" <- w249
            n163 = property on="Panel1" class="SubPnl"("Visible"=FALSE, "AllowBDOpen"=FALSE ("Allow User to Open Diagram"), "MakePanelTransparent"=FALSE ("Panel Transparent")) -> ()  [unwired: 2 in, 2 out]
          }
          frame #1 {
            # "Open references"
            n164 = call <vilib>:"Initialize Mouse.vi"() -> ("device ID"=→"DeviceID":refnum<k1>)  [unwired: 10 in, 1 out]
            n165 = control-ref of="Btn_Exit"() -> (w287:refnum<vi>)
            n166 = control-ref of="Btn_Mode"() -> (w286:refnum<vi>)
            n167 = control-ref of="Btn_Process"() -> (w285:refnum<vi>)
            n168 = control-ref of="Btn_Base"() -> (w284:refnum<vi>)
            n169 = control-ref of="Btn_Order"() -> (w283:refnum<vi>)
            n170 = control-ref of="Btn_Manual"() -> (w274:refnum<vi>)
            n171 = control-ref of="Btn_Logs"() -> (w277:refnum<vi>)
            n172 = control-ref of="Btn_Results"() -> (w273:refnum<vi>)
            n173 = control-ref of="Btn_Accept"() -> (w276:refnum<vi>)
            n174 = control-ref of="Btn_Reject"() -> (w275:refnum<vi>)
            n175 = control-ref of="Btn_Start"() -> (w282:refnum<vi>)
            n176 = control-ref of="Btn_Stop"() -> (w281:refnum<vi>)
            n177 = control-ref of="Btn_Next"() -> (w280:refnum<vi>)
            n178 = control-ref of="Btn_Pause"() -> (w272:refnum<vi>)
            n179 = control-ref of="Btn_Lock"() -> (w271:refnum<vi>)
            n180 = control-ref of="Btn_ManualView"() -> (w270:refnum<vi>)
            n181 = control-ref of="Btn_DoorLock"() -> (w269:refnum<vi>)
            n182 = control-ref of="Btn_Scan"() -> (w268:refnum<vi>)
            n183 = control-ref of="Btn_SelectPlate"() -> (w267:refnum<vi>)
            n184 = control-ref of="Btn_ScannerGui"() -> (w266:refnum<vi>)
            n185 = control-ref of="Btn_Stats"() -> (w265:refnum<vi>)
            n186 = Build Array(w287, w286, w285, w284, w283, w274, w277, w273, w276, w275, w282, w281, w280, w272, w271, w270, w269, w268, w267, w266, w265) -> (w279:refnum<vi>[])
            "Btns" <- w279
            n187 = call "MainGui.Buttons.Show.vi"("Show (F)"=TRUE, "Btns"=w279) -> ()  [unwired: 1 in]
            "MainPanelViRef" <- refnum<vi> refnum ("MainPanelViRef")
          }
          frame #2 {
            n188 = global read "ApplicationGlobal.vi" "Unlock"() -> (w290:bool)
            n189 = property on="Btn_Lock" class="Bool (strict)"("Value"=w290) -> ()  [unwired: 2 in, 2 out]
            n190 = Select(t=T6."Enabled" ("Disabled"), s=w290, f=T6."Disabled and Grayed Out" ("Disabled")) -> (s? t:f=w291:T6)
            n191 = property on="IgnoreResults" class="Bool (strict)"("DisabledEnum"=w291) -> (error out=w293:errorcluster)  [unwired: 2 in, 1 out]
            n192 = property on="IgnoreImages" class="Bool (strict)"(error in=w293, "DisabledEnum"=w291) -> (error out=w292:errorcluster)  [unwired: 1 in, 1 out]
            n193 = property on="Service" class="Bool (strict)"(error in=w292, "DisabledEnum"=w291) -> ()  [unwired: 1 in, 2 out]
          }
          frame #3 {
            # "Set default states before translation"
            n194 = Unbundle By Name(T13 {"Msg"=enum."Initializing", "Arguments"=[], "BgColor"=16744448, "TxtColor"=16448250, "Blink"=FALSE} ("UsrMsg")) -> ("BgColor"=w301:u32, "TxtColor"=w300:u32, "Blink"=w299:bool, "Msg"=w298:T7, "Arguments"=w297:variant[])
            n195 = call "Translator.Translate.Status (NoError).vi"("Arguments"=w297, "msg"=w298) -> ("Translated Msg"=w296:string)  [unwired: 9 in]
            n196 = property on="StatusMsg" class="Str"("Text.BGColor"=w301, "Text.TextColor"=w300, "Blinking"=w299, "Value"=w296) -> ()  [unwired: 2 in, 2 out]
          }
          frame #4 {
            # "Init Top Bar"
            n197 = global read "ApplicationGlobal.vi" "StationNo"() -> (w303:i32)
            n198 = global read "ApplicationGlobal.vi" "AppName"() -> (w305:string)
            n199 = global read "ApplicationGlobal.vi" "AppVer"() -> (w304:string)
            n200 = property on="TopBarTab" class="TabCtl (strict)"("Value"=0, "Page Labels Display Visible?"=FALSE) -> ()  [unwired: 2 in, 2 out]
            n201 = Format Into String(format string="%d. %s %s", w303, w305, w304) -> (resulting string=w318:string)  [unwired: 2 in, 1 out]
            n202 = global read "Config.Global.vi" "LogsOptions"() -> (w315:T2)
            n203 = property class="App"() -> ("App.Kind"=w308:T14)  [unwired: 2 in, 2 out]
            n204 = global read "Config.Global.vi" "Touchpanel"() -> (w321:bool)
            n205 = Not Equal?(x=w308, y=T14."Run Time System") -> (x != y?=w306:bool)
            n206 = local write "EventModeOptions"(w315) -> ()
            n207 = property on="_loop" class="Ring (strict)"("Visible"=w306) -> ()  [unwired: 2 in, 2 out]
            n208 = Bundle By Name(cluster="TopBar", "~touchpanel"=w321, "_ver"=w318) -> (w320:T4)
            n209 = local write "TopBar"(w320) -> ()
            n210 = property on="ErrMsg" class="MCListbox (strict)"("ItemNames"=string[][] [] ("Item Names"), "EditPos"=T16 {"Row"=-2, "Column"=-2} ("Edit Position"), "SelColor"=u32 16777216, "TopLeft"=T15 {"Row"=0, "Column"=0} ("Top Left Visible Cell")) -> ()  [unwired: 2 in, 2 out]
            "ErrMsg" <- -1 ("ErrMsg")
          }
          frame #5 {
            n211 = global read "Translator.Global.vi" "Translations.Source"() -> (w322:string[])
            n212 = global read "Translator.Global.vi" "Translations.Level"() -> (w323:string[])
            n213 = property on="Level" class="Ring (strict)"("Strings []"=w323) -> ()  [unwired: 2 in, 2 out]
            n214 = property on="Source" class="Ring (strict)"("Strings []"=w322) -> ()  [unwired: 2 in, 2 out]
          }
          frame #6 {
            # "Translate VI"
            n215 = global read "Translator.Global.vi" "Flag"() -> (w327:picture)
            n216 = global read "Config.Global.vi" "UserSets"() -> (w328:T31)
            n217 = call "Translator.TranslateThis.Init.vi"("error in"=w329) -> ("error out"=w324:errorcluster)  [unwired: 10 in]
            n218 = property on="_flag" class="Pict"("Value"=w327) -> ()  [unwired: 2 in, 2 out]
            n219 = Unbundle By Name(w328) -> ("Test"=w326:T32)
            n220 = local write "TestOptions"(w326) -> ()
          }
          frame #7 {
            # "Set default states after translation"
            n221 = disable-structure shown="Disabled" {
              frame Disabled {
                n222 = while {
                  stop <- w333 stop-if-true
                  n223 = global read "ApplicationGlobal.vi" "AppLaunched"() -> (w333:bool)
                  n224 = Wait (ms)(milliseconds to wait=u32 50) -> ()  [unwired: 1 out]
                }
              }
              frame Enabled {
              }
            }
            n225 = local read "Btns"() -> (w330:refnum<vi>[])
            n226 = call "MainGui.Buttons.Show.vi"("Show (F)"=FALSE, "Btns"=w330) -> ()  [unwired: 1 in]
          }
        }
      }
      frame "destructor" {
        # "Application shutdown actions"
        n227 = stacked-sequence {
          tunnel: w336 -> [_ _ _ _ _ _ w359 _]
          tunnel: [_ _ _ _ _ _ w358 _] -> w335
          frame #0 {
            # "Restore controls to default state"
            # "Set default states before translation"
            n228 = property on="Pane" class="Pane"("PaneColor"=u32 16777226) -> ()  [unwired: 2 in, 2 out]
            n229 = invoke on="Panel1" class="SubPnl" method="Remove VI"() -> ()  [unwired: 3 in, 3 out]
            n230 = property on="TopBarTab" class="TabCtl (strict)"("Value"=0, "Page Labels Display Visible?"=TRUE) -> ()  [unwired: 2 in, 2 out]
            n231 = Unbundle By Name(T13 {"Msg"=enum."Quitting", "Arguments"=[], "BgColor"=16744448, "TxtColor"=16448250, "Blink"=FALSE} ("UsrMsg")) -> ("BgColor"=w344:u32, "TxtColor"=w343:u32, "Blink"=w342:bool, "Msg"=w341:T7, "Arguments"=w340:variant[])
            n232 = local read "Btns"() -> (w350:refnum<vi>[])
            n233 = call "MainGui.Buttons.Show.vi"("Show (F)"=TRUE, "Btns"=w350) -> ()  [unwired: 1 in]
            n234 = call "Translator.Translate.Status (NoError).vi"("Arguments"=w340, "msg"=w341) -> ("Translated Msg"=w339:string)  [unwired: 9 in]
            n235 = property on="Panel1" class="SubPnl"("Visible"=FALSE) -> ()  [unwired: 2 in, 2 out]
            n236 = property on="StatusMsg" class="Str"("Text.BGColor"=w344, "Text.TextColor"=w343, "Blinking"=w342, "Value"=w339) -> ()  [unwired: 2 in, 2 out]
            n237 = call "Translator.Translate.Status (NoError).vi"("msg"=Translator.Message."Quitting") -> ("Translated Msg"=w346:string)  [unwired: 10 in]
            n238 = property class="VI"("Front Panel.ShowMenuBar"=FALSE ("Front Panel Window:Show Menu Bar")) -> ()  [unwired: 2 in, 2 out]
            n239 = call "Wait.Gui.Open.vi"("Msg"=w346) -> ()  [unwired: 10 in, 1 out]
          }
          frame #1 {
            w353 = TRUE ("Abort")
            # "Close references"
            n240 = global write "Keyence.Global.vi" "Keyence.Abort"(w353) -> ()
            n241 = global write "FestoCPX.Global.vi" "FestoCPX.Abort"(w353) -> ()
            n242 = global write "V7310.Global.vi" "Laser.Abort"(w353) -> ()
            n243 = local read "DeviceID"() -> (w354:refnum<k1>)
            n244 = local read "Btns"() -> (w355:refnum<vi>[])
            n245 = Close Reference(reference=w355) -> ()  [unwired: 1 in, 1 out]
            n246 = call-poly <vilib>:"Close Input Device.vi"("device ID"=w354) -> ()  [unwired: 9 in, 1 out]
          }
          frame #2 {
            # "Close sequence loop"
            n247 = disable-structure shown="Disabled" {
              frame Disabled {
                n248 = call "Sequence-Kill.vi"() -> ()  [unwired: 11 in, 1 out]
              }
              frame Enabled {
              }
            }
          }
          frame #3 {
            # "Close station loop"
            n249 = call "Station-Kill.vi"() -> ()  [unwired: 11 in, 1 out]
          }
          frame #4 {
            # "close database loops"
            n250 = call "Database.Main-Kill.vi"() -> ()  [unwired: 11 in, 1 out]
          }
          frame #5 {
            n251 = call "Keyence.Main-Destructor.vi"("Idx"=0) -> ()  [unwired: 10 in, 1 out]
            n252 = call "Keyence.Main-Destructor.vi"("Idx"=1) -> ()  [unwired: 10 in, 1 out]
            n253 = call "FestoCPX-Kill.vi"() -> ()  [unwired: 11 in, 1 out]
            n254 = call "V7310.Main-Destructor.vi"() -> ()  [unwired: 11 in, 1 out]
          }
          frame #6 {
            # "Translate VI back to English"
            n255 = call "Translator.TranslateThis.Exit.vi"("error in"=w359) -> ("error out"=w358:errorcluster)  [unwired: 10 in]
          }
          frame #7 {
            # "Close all other loops"
            n256 = global write "User.Global.vi" "UserLoggedIn"(-1 ("UserLoggedIn")) -> ()
            n257 = global write "User.Global.vi" "Guru"(FALSE ("Guru")) -> ()
            n258 = global write "User.Global.vi" "UserLevel"(User.Level."-" ("UserLevel")) -> ()
            n259 = Unbundle By Name(T13 {"Msg"=enum."Quitting", "Arguments"=[], "BgColor"=16777225, "TxtColor"=0, "Blink"=FALSE} ("UsrMsg")) -> ("BgColor"=w366:u32, "TxtColor"=w365:u32, "Blink"=w364:bool, "Msg"=w363:T7, "Arguments"=w362:variant[])
            n260 = call "citTemplate.writeQueue.vi"("High priority (F)"=TRUE, "data in"="destructor") -> ()  [unwired: 13 in, 1 out]
            n261 = call "Translator.Translate.Status (NoError).vi"("Arguments"=w362, "msg"=w363) -> ("Translated Msg"=w361:string)  [unwired: 9 in]
            n262 = property on="StatusMsg" class="Str"("Text.BGColor"=w366, "Text.TextColor"=w365, "Blinking"=w364, "Value"=w361) -> ()  [unwired: 2 in, 2 out]
            n263 = property on="Panel1" class="SubPnl"("Visible"=TRUE) -> ()  [unwired: 2 in, 2 out]
          }
        }
      }
      frame "--- MainGui ---" {
        w377 = EventLog.EventSource."Gui" ("Event source")
        # "--> Handle error here..."
        # "Error handler"
        n264 = Unflatten From String(type=T18 {"ts"=timestamp(0 s since 1904-01-01), "src"=enum."All", "instance"=0, "action"="", "error"={"status"=FALSE, "code"=0, "source"=""}, "unconfirmed"=FALSE} ("ErrData"), binary string=w382, error in (no error)=w384) -> (value=w376:T18, error out=w375:errorcluster)  [unwired: 3 out]
        n265 = disable-structure shown="Disabled" {
          disable-tunnel: w381 -> [w390 _]
          frame Disabled {
            n266 = global read "ApplicationGlobal.vi" "Quitting"() -> (w391:bool)
            n267 = case shown="False" w391 {
              tunnel: w390 -> [w392 _]
              frame False {
                n268 = call "citTemplate.clearQueue.vi"("event in"=w392) -> ()  [unwired: 13 in, 2 out]
              }
              frame True {
              }
            }
          }
          frame Enabled {
          }
        }
        n269 = call "ErrorHandling.Fglb.Add.vi"("Event source"=w377, "error in (no error)"=w375, "Error in"=w376) -> ("error out"=w379:errorcluster, "changed?"=w378:bool)  [unwired: 7 in]
        n270 = case shown="True" w378 {
          tunnel: [w385 w389] -> w374
          tunnel: w376 -> [_ w388]
          tunnel: w379 -> [w385 w387]
          tunnel: w377 -> [_ w386]
          frame False {
          }
          frame True {
            n271 = call "EventLog.New(error).vi"("Source (All)"=w386, "error in"=w387, "ErrData"=w388) -> ("error out"=w389:errorcluster)  [unwired: 8 in]
          }
        }
        n272 = call <vilib>:"Clear Errors.vi"("error in (no error)"=w374) -> ("error out"=w373:errorcluster)  [unwired: 5 in, 1 out]
      }
      frame "Error.Update" {
        n273 = call "ErrorHandling.Fglb.Check.vi"("error in (no error)"=w396) -> ("error out"=w395:errorcluster, "changed?"=w394:bool)  [unwired: 9 in]
        n274 = case shown="True" w394 {
          tunnel: [w398 w404] -> w397
          tunnel: w395 -> [w398 w406]
          tunnel: w393 -> [_ w401]
          frame False {
          }
          frame True {
            n275 = call "ErrorHandling.Fglb.Get.vi"("error in (no error)"=w406) -> ("error out"=w404:errorcluster, "Errors"=w407:T18[], "unconfirmed?"=w403:bool)  [unwired: 8 in]
            n276 = case shown="Default" w401 {
              tunnel: [enum32{"Status", "Manual", "Logs", "Error"}."Status" ("TopBarTab") enum32{"Status", "Manual", "Logs", "Error"}."Manual" ("TopBarTab") enum32{"Status", "Manual", "Logs", "Error"}."Logs" ("TopBarTab")] -> w400
              frame Default {
              }
              frame "Manual" {
              }
              frame "Logs" {
              }
            }
            n277 = Array Size(array=w407) -> (size(s)=w408:i32)
            n278 = Greater Than 0?(x=w408) -> (x > 0?=w402:bool)
            n279 = for {
              tunnel: w407 -> [w424] mode=indexing
              tunnel: [w419] -> w412 mode=indexing
              (unwired) EventLog.EventSource."All" ("src")
              n280 = Unbundle By Name(w424) -> ("src"=w418:T19, "ts"=w423:timestamp, "error.source"=w417:string)
              n281 = call "EventLog.FormatErrorMessage.vi"("Error string in"=w417) -> ("Error string out"=w416:string)
              n282 = Format Into String(w418) -> (resulting string=w420:string)  [unwired: 3 in, 1 out]
              n283 = Format Date/Time String(time format string (%c)="%H:%M:%S", seconds (now)=w423) -> (date/time string=w421:string)  [unwired: 1 in]
              n284 = Build Array(w420, w421, w416) -> (w419:string[])
            }
            n285 = Select(t=enum32{"Status", "Manual", "Logs", "Error"}."Error" ("TopBarTab"), s=w403, f=w400) -> (s? t:f=w405:enum32{"Status", "Manual", "Logs", "Error"})
            n286 = property on="Btn_ShowErr" class="Bool (strict)"("Visible"=w402, "Value"=w403) -> ()  [unwired: 2 in, 2 out]
            n287 = property on="TopBarTab" class="TabCtl (strict)"("Value"=w405) -> ()  [unwired: 2 in, 2 out]
            n288 = global write "ApplicationGlobal.vi" "UnconfirmedError"(w403) -> ()
            n289 = property on="ErrMsg" class="MCListbox (strict)"("ItemNames"=w412, "Value"=-1 ("ErrMsg"), "EditPos"=T16 {"Row"=-2, "Column"=-2} ("Edit Position"), "TopLeft"=T15 {"Row"=0, "Column"=0} ("Top Left Visible Cell")) -> ()  [unwired: 2 in, 2 out]
          }
        }
      }
      frame "Error.Confirm" {
        n290 = call "ErrorHandling.Fglb.Confirm.vi"("error in (no error)"=w426) -> ("error out"=w425:errorcluster)  [unwired: 10 in]
      }
      frame "Buttons.Update" {
        # "Update buttons"
        n291 = local read "Panel"() -> (w429:refnum<vi>)
        n292 = property class="Pnl"(reference=w429, error in=w434, "DeferPanUpdts"=TRUE ("Defer Panel Updates")) -> (reference out=w430:refnum<vi>, error out=w431:errorcluster)
        n293 = local read "Btns"() -> (w438:refnum<vi>[])
        n294 = call "MainGui.Buttons.Update.vi"("Btns"=w438, "error in (no error)"=w431, "Mode"=w437) -> ("error out"=w433:errorcluster)  [unwired: 8 in]
        n295 = call <vilib>:"Clear Errors.vi"("error in (no error)"=w433) -> ("error out"=w428:errorcluster)  [unwired: 5 in, 1 out]
        n296 = property class="Pnl"(reference=w430, error in=w428, "DeferPanUpdts"=FALSE ("Defer Panel Updates")) -> (error out=w432:errorcluster)  [unwired: 1 out]
      }
      frame "Mode.Select" {
        # "Select applpication mode - prepare panels to display specific GUI"
        n297 = Unflatten From String(type=Sequence.MainMode."Process" ("Mode"), binary string=w444, error in (no error)=w445) -> (value=w440:T8, error out=w442:errorcluster)  [unwired: 2 in, 1 out]
        n298 = stacked-sequence {
          tunnel: w442 -> [_ w468 _]
          tunnel: [_ w466 _] -> w441
          tunnel: w440 -> [w449 w467 _]
          tunnel: w439 -> [_ w463 _]
          frame #0 {
            n299 = global read "Translator.Global.vi" "Translations.GuiMode"() -> (w451:string[])
            n300 = local write "Btn_Mode"(FALSE ("Btn_Mode")) -> ()
            n301 = Index Array(array=w451, index=w449) -> (element=w446:string)
            n302 = property on="ErrMsg" class="MCListbox (strict)"() -> ("ItemNames"=w453:string[][])  [unwired: 2 in, 2 out]
            n303 = property on="~ModeInUse" class="Bool"("BoolText.Text"=w446) -> ()  [unwired: 2 in, 2 out]
            n304 = Empty Array?(array=w453) -> (empty?=w452:bool)
            n305 = case shown="\"Manual\"" w449 {
              tunnel: [enum32{"Status", "Manual", "Logs", "Error"}."Status" ("TopBarTab") enum32{"Status", "Manual", "Logs", "Error"}."Manual" ("TopBarTab") enum32{"Status", "Manual", "Logs", "Error"}."Logs" ("TopBarTab")] -> w448
              frame Default {
              }
              frame "Manual" {
              }
              frame "Logs" {
              }
            }
            n306 = property on="Panel1" class="SubPnl"("Visible"=FALSE) -> ()  [unwired: 2 in, 2 out]
            n307 = Select(t=w448, s=w452, f=enum32{"Status", "Manual", "Logs", "Error"}."Error" ("TopBarTab")) -> (s? t:f=w454:enum32{"Status", "Manual", "Logs", "Error"})
            n308 = property on="TopBarTab" class="TabCtl (strict)"("Value"=w454) -> ()  [unwired: 2 in, 2 out]
          }
          frame #1 {
            n309 = invoke on="Panel1" class="SubPnl" method="Remove VI"(error in=w468) -> (error out=w462:errorcluster)  [unwired: 2 in, 2 out]
            n310 = case shown="Default" w463 {
              tunnel: w462 -> [w470]
              tunnel: [w470] -> w461
              frame Default {
              }
            }
            n311 = case shown="\"Logs\"" w467 {
              tunnel: [w480 w484 w488 w492 w496 w500 w504 w508] -> w469
              tunnel: [T6."Disabled" ("Disabled") T6."Disabled" ("Disabled") T6."Disabled" ("Disabled") T6."Disabled" ("Disabled") T6."Disabled" ("Disabled") T6."Disabled" ("Disabled") T6."Disabled" ("Disabled") T6."Disabled" ("Disabled")] -> w465
              tunnel: w461 -> [w478 w482 w486 w490 w494 w498 w502 w506]
              tunnel: [w478 w482 w486 w490 w494 w498 w502 w506] -> w464
              tunnel: [u32 16777226 u32 13816530 u32 13816530 u32 13816530 u32 13816530 u32 13816530 u32 13816530 u32 16777226] -> w459
              frame "Process" {
                n312 = global read "ApplicationGlobal.vi" "GuiRef.TestSteps"() -> (w480:refnum<vi>)
              }
              frame "Base" {
                n313 = global read "ApplicationGlobal.vi" "GuiRef.Base"() -> (w484:refnum<vi>)
              }
              frame "DMC Config" {
                n314 = global read "ApplicationGlobal.vi" "GuiRef.DMCConfig"() -> (w488:refnum<vi>)
              }
              frame "Logs" {
                n315 = global read "ApplicationGlobal.vi" "GuiRef.Logs"() -> (w492:refnum<vi>)
              }
              frame "Results" {
                n316 = global read "ApplicationGlobal.vi" "GuiRef.Results"() -> (w496:refnum<vi>)
              }
              frame "Stats" {
                n317 = global read "ApplicationGlobal.vi" "GuiRef.Stats"() -> (w500:refnum<vi>)
              }
              frame "Manual" {
                n318 = global read "ApplicationGlobal.vi" "GuiRef.Daq"() -> (w504:refnum<vi>)
              }
              frame "Order" {
                n319 = global read "ApplicationGlobal.vi" "GuiRef.ChangeOver"() -> (w508:refnum<vi>)
              }
            }
            n320 = Not A Number/Path/Refnum?(number/path/refnum=w469) -> (NaN/Path/Refnum?=w460:bool)
            n321 = property on="StatusMsg" class="Str"("DisabledEnum"=w465) -> ()  [unwired: 2 in, 2 out]
            n322 = case shown="False" w460 {
              tunnel: w464 -> [w474 w476]
              tunnel: [w475 w476] -> w466
              tunnel: w469 -> [w473 _]
              tunnel: [w471 _] -> _
              frame False {
                n323 = invoke class="VI" method="FP.Close"(reference=w473) -> (reference out=w472:refnum<vi>, error out=w471:errorcluster)  [unwired: 2 in, 1 out]
                n324 = invoke on="Panel1" class="SubPanel" method="Insert VI"(error in=w474, "VI Ref"=w472) -> (error out=w475:errorcluster)  [unwired: 2 in, 3 out]
              }
              frame True {
              }
            }
            n325 = property on="Pane" class="Pane"("PaneColor"=w459) -> ()  [unwired: 2 in, 2 out]
          }
          frame #2 {
            n326 = property on="Panel1" class="SubPnl"("Visible"=TRUE) -> ()  [unwired: 2 in, 2 out]
          }
        }
        n327 = call "MainGui-ModeSelectSeq.vi"() -> ()  [unwired: 11 in, 1 out]
      }
      frame "Mode.Select.Seq" {
        n328 = global read "Station.Global.vi" "Station"() -> (w517:T24)
        n329 = global read "Config.Global.vi" "UserSets"() -> (w511:T31)
        n330 = Unbundle By Name(w517) -> ("State"=w513:T25)
        n331 = case shown="\"Manual\"" w516 {
          selector: w516 -> [w520 w522]
          tunnel: w511 -> [w521 w524]
          tunnel: [w519 w523] -> w514
          tunnel: w513 -> [_ _]
          tunnel: "TestOptions" -> [w518 _]
          frame "Manual" {
            n332 = Bundle By Name(cluster=w521, "GuiMode"=w520, "Test"=w518) -> (w519:T31)
          }
          frame Default {
            n333 = Bundle By Name(cluster=w524, "GuiMode"=w522) -> (w523:T31)
          }
        }
        n334 = call "Station-ModeSelect.vi"("error in (no error)"=w515, "SeqOptions"=w514) -> ("error out"=w510:errorcluster)  [unwired: 9 in]
        n335 = global write "Config.Global.vi" "UserSets"(w514) -> ()
      }
      frame "Status.Update" {
        # "Update status of running sequence"
        n336 = Unflatten From String(type=T13 {"Msg"=enum."-", "Arguments"=[], "BgColor"=0, "TxtColor"=0, "Blink"=FALSE} ("UsrMsg"), binary string=w537, error in (no error)=w538) -> (value=w529:T13, error out=w527:errorcluster)  [unwired: 2 in, 1 out]
        n337 = while {
          tunnel: w529 -> [w544]
          tunnel: w527 -> [w542]
          shift-right: [w543] -> w528
          shift-left: _ -> [w540]
          stop <- TRUE stop-if-true
          n338 = case shown="Error" w542 {
            tunnel: [w545 w546] -> w543
            tunnel: w544 -> [w545 _]
            tunnel: w540 -> [_ w546]
            frame No Error {
            }
            frame Error {
            }
          }
        }
        n339 = Unbundle By Name(w528) -> ("BgColor"=w534:u32, "TxtColor"=w533:u32, "Blink"=w532:bool, "Msg"=w525:T7, "Arguments"=w531:variant[])
        n340 = call <vilib>:"Clear Errors.vi"("error in (no error)"=w527) -> ("error out"=w530:errorcluster)  [unwired: 5 in, 1 out]
        n341 = call "Translator.Translate.Status (NoError).vi"("Arguments"=w531, "msg"=w525) -> ("Translated Msg"=→"StatusMsg":string)  [unwired: 9 in]
        n342 = property on="StatusMsg" class="Str"(error in=w530, "Text.BGColor"=w534, "Text.TextColor"=w533, "Blinking"=w532) -> (error out=w535:errorcluster)  [unwired: 1 in, 1 out]
      }
      frame "TopBar.Update" {
        n343 = stacked-sequence {
          frame #0 {
            n344 = call "Database.Main-GetTime.vi"() -> ("TS"=w549:timestamp)  [unwired: 1 in]
            n345 = global read "Keyence.Global.vi" "OrderScanner.Status"() -> (w553:T36)
            n346 = global read "Keyence.Global.vi" "ProdScanner.Status"() -> (w559:T36)
            n347 = global read "FestoCPX.Global.vi" "FestoCPX.Status"() -> (w567:T37)
            n348 = global read "V7310.Global.vi" "Laser.Status"() -> (w563:T38)
            n349 = global read "Database.Global.vi" "DB.Status"() -> (w556:T42)
            n350 = Unbundle By Name(w567) -> ("State"=w566:T22)
            n351 = Unbundle By Name(w563) -> ("State"=w564:T21)
            n352 = Unbundle By Name(w559) -> ("State"=w560:T20)
            n353 = Unbundle By Name(w553) -> ("State"=w552:T20)
            n354 = Unbundle By Name(w556) -> ("Run"=w555:bool)
            n355 = Format Date/Time String(time format string (%c)="%Y-%m-%d %H:%M:%S%1u", seconds (now)=w549) -> (date/time string=w570:string)  [unwired: 1 in]
            n356 = Equal?(x=w566, y=FestoCPX.State."Run") -> (x = y?=w550:bool)
            n357 = Greater Or Equal?(x=w564, y=V7310.Data.Status.State."Idle") -> (x >= y?=w561:bool)
            n358 = Greater Or Equal?(x=w560, y=Keyence.Data.Status.State."Idle") -> (x >= y?=w558:bool)
            n359 = Greater Or Equal?(x=w552, y=Keyence.Data.Status.State."Idle") -> (x >= y?=w551:bool)
            n360 = local read "TopBar"() -> (w572:T4)
            n361 = Bundle By Name(cluster=w572, "time"=w570, "DB"=w555, "CPX"=w550, "LSR"=w561, "SCAN"=w558, "SCAN 2"=w551) -> (w569:T4)
            n362 = local write "TopBar"(w569) -> ()
            n363 = Unbundle By Name(w569) -> ("~touchpanel"=w571:T5)
            n364 = global write "Config.Global.vi" "Touchpanel"(w571) -> ()
          }
        }
      }
    }
    n365 = call "citTemplate.ErrorEventPass.vi"("error in"=w3, "action of error"=w6, "event in"=w10) -> ("error out"=w7:errorcluster)  [unwired: 2 in, 6 out]
  }
  n366 = disable-structure shown="Disabled" {
    frame Disabled {
      (unwired) MainGui.ButtonType."Lock" ("Button")
      (unwired) Sequence.MainMode."Process" ("Mode")
      # "Put important VIs here..."
      n367 = call "citTemplate.clearQueue.vi"() -> ()  [unwired: 14 in, 2 out]
      n368 = call "citTemplate.writeQueue.vi"() -> ()  [unwired: 15 in, 1 out]
      n369 = call "citTemplate.writeQueueWithAck.vi"() -> ()  [unwired: 13 in, 3 out]
      n370 = call "citTemplate.ErrorEventPass.vi"() -> ()  [unwired: 11 in, 1 out]
      n371 = Flatten To String() -> ()  [unwired: 4 in, 3 out]
      n372 = Unflatten From String() -> ()  [unwired: 5 in, 3 out]
      n373 = call "MainGui-Error.vi"() -> ()  [unwired: 11 in, 1 out]
      n374 = call "MainGui-Reboot.vi"() -> ()  [unwired: 11 in, 1 out]
      n375 = call "MainGui-SeqResultStatus.vi"() -> ()  [unwired: 11 in, 1 out]
      n376 = call "MainGui-ModeSelect.vi"() -> ()  [unwired: 11 in, 1 out]
      n377 = call "MainGui-ButtonsUpdate.vi"() -> ()  [unwired: 11 in, 1 out]
      n378 = call "MainGui-ModeSelectSeq.vi"() -> ()  [unwired: 11 in, 1 out]
      n379 = call "Translator.TranslateThis.Init.vi"() -> ()  [unwired: 11 in, 1 out]
      n380 = call "Translator.TranslateThis.Exit.vi"() -> ()  [unwired: 11 in, 1 out]
      n381 = call "Daq.Gui.vi"() -> ()  [unwired: 12 in]
      n382 = call "TestStepsGui.vi"() -> ()  [unwired: 12 in]
      n383 = call "MainGui.Buttons.Update.vi"() -> ()  [unwired: 11 in, 1 out]
    }
    frame Enabled {
    }
  }
  n384 = disable-structure shown="Disabled" {
    frame Disabled {
      n385 = local read "BlinkIndicator"() -> (w581:bool)
      n386 = local read "RefNoTimer"() -> (w579:timestamp)
      n387 = Get Date/Time In Seconds() -> (seconds since 1Jan1904=w574:timestamp)
      n388 = Greater?(x=w574, y=w579) -> (0:w580:bool)
      n389 = Select(t=2.0 ("y"), s=w581, f=0.5) -> (s? t:f=w577:dbl)
      n390 = case shown="False" w580 {
        tunnel: [w582 w588] -> w573
        tunnel: w574 -> [_ w587]
        tunnel: [w583 w586] -> w575
        tunnel: w577 -> [_ w585]
        tunnel: w581 -> [w583 w584]
        tunnel: w579 -> [w582 _]
        frame False {
        }
        frame True {
          n391 = Not(x=w584) -> (.not. x?=w586:bool)
          n392 = Add(x=w587, y=w585) -> (x+y=w588:timestamp)
        }
      }
      "RefNoTimer" <- w573
      "BlinkIndicator" <- w575
    }
    frame Enabled {
    }
  }
